vi "Get ID from Queue.vi"(8 "error in (no error)":errorcluster, 10 "uService Queue":refnum<class "Message Enqueuer.lvclass">, 11 "uService List in":refnum<class "uService List.lvclass">) -> (0 "error out":errorcluster, 2 "ID out":string, 3 "uService List out":refnum<class "uService List.lvclass">)   [LabVIEW 2026, in "TALOS.lvlib" / "Classes.lvlib" / "uService List.lvclass"]
uses:
  uService List.lvclass
  builds/Actor Framework PPL/Actor Framework.lvlibp/1abvi3w/vi.lib/ActorFramework/Message Enqueuer/Message Enqueuer.lvclass
  uService List.lvclass/uService List.ctl
  Ancestor/Ancestor/Ancestor.lvclass/Ancestor.ctl
  FGV/Error Memory/Get Error Description.vi
  Support VIs/Get PC name.vi
  Ancestor/Ancestor/Read ID.vi
  Support VIs/Get Class Name.vi
  <vilib>/Utility/error.llb/Clear Errors.vi
  FGV/Error Memory/Error Memory Core.vi
  <vilib>/AdvancedString/Delimited String to 1D String Array.vi
  <vilib>/AdvancedString/Delimited String to 1D String Array (string).vi
  Support VIs/Circus Root Path.vi
  FGV/Error Memory/Error Crt Lvl checker.vi
  FGV/Error Memory/Error Memory Core.vi/40c8088d-b597-4017-91af-faa98e00292e.vi
  FGV/Error Memory/Error Memory Core.vi/d4a3ab98-063c-4e44-b43d-fbdcfe6c2be2.vi
  Support VIs/Global Memory.vi
  <vilib>/Utility/LVClass/Get LV Class Name.vi
  Support VIs/Is in Packed Library.vi
  Support VIs/TALOS Root path.vi
  Support VIs/Read CSV worksheet.vi
  Support VIs/Global Constants.vi
  <vilib>/Utility/error.llb/General Error Handler.vi
  Ancestor/Ancestor/Ancestor.lvclass
  <vilib>/Comparison/Equal/Equal Functor/Equal Functor.lvclass
  TALOS.lvlib
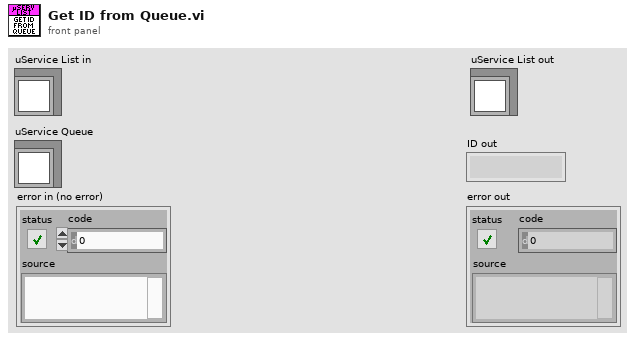
[diagram p1: front panel]
types:
  T1 = typedef "TALOS.lvlib/Classes.lvlib/uService List.lvclass/uService Properties.ctl" = cluster{"uService Queue":refnum<class "Message Enqueuer.lvclass">, "Last Pat":timestamp, "Online":bool, "Vi Ref":refnum<vi>, "Class name":string, "GUI":bool, "FP Items Refs Map":map{string, refnum<vi>}, "Remote GUI":bool, "Remote Window":refnum<vi>}
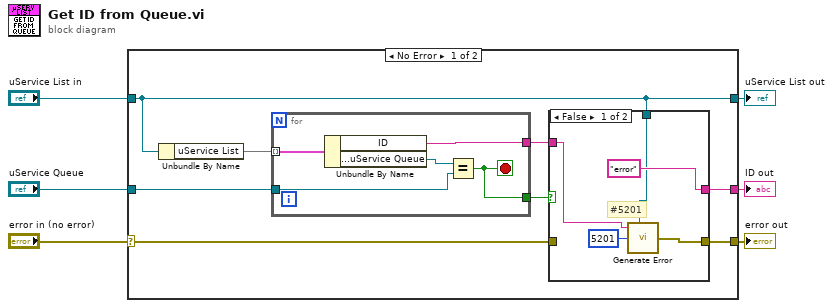
[diagram p0: block diagram]
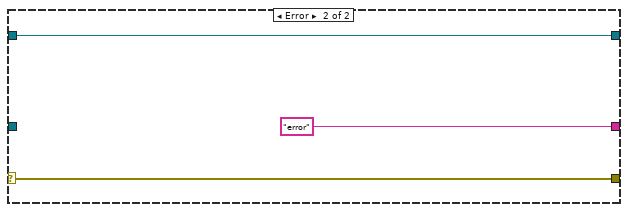
[diagram p3: hidden frame]
diagram:
  n1 = case shown="No Error" "error in (no error)" {
    selector: "error in (no error)" -> [w10 w27]
    tunnel: "uService List in" -> [w7 w29]
    tunnel: [w7 w29] -> w4
    tunnel: "uService Queue" -> [w13 _]
    tunnel: [w8 "error"] -> w2
    tunnel: [w9 w27] -> w1
    frame No Error {
      n2 = Unbundle By Name(w7) -> ("uService List"=w14:map{string, T1})
      n3 = for {
        tunnel: w14 -> [w26] mode=indexing
        tunnel: [w25] -> w12
        tunnel: w13 -> [w23]
        tunnel: [w22] -> w11
        stop <- w22 stop-if-true
        n4 = Unbundle By Name(w26) -> ("ID"=w25:string, "uService Properties.uService Queue"=w24:refnum<class "Message Enqueuer.lvclass">)
        n5 = Equal?(x=w24, y=w23) -> (x = y?=w22:bool)
      }
      n6 = case shown="False" w11 {
        tunnel: ["error" ("ID") w21] -> w8
        tunnel: w12 -> [w15 w21]
        tunnel: [w17 w20] -> w9
        tunnel: w10 -> [_ w20]
        tunnel: w7 -> [w16 _]
        frame False {
          # "#5201"
          n7 = call "Generate Error.vi"("Optional String"=w15, "Class"=w16, "Error Code"=5201) -> ("error out"=w17:errorcluster)  [unwired: 4 in]
        }
        frame True {
        }
      }
    }
    frame Error {
    }
  }
  "error out" <- w1
  "ID out" <- w2
  "uService List out" <- w4
